vi "Update State.vi"(10 "Async Auth State":T1, 11 "Async Authorization in":refnum<class "Async Authorization.lvclass">) -> (3 "Async Authorization out":refnum<class "Async Authorization.lvclass">)   [LabVIEW 2020, in "OAuth2.lvlib" / "Async Authorization.lvclass"]
uses:
  Async Authorization.lvclass
  Async Auth State.ctl
  Async Authorization.lvclass/Async Authorization.ctl
  OAuth2.lvlib
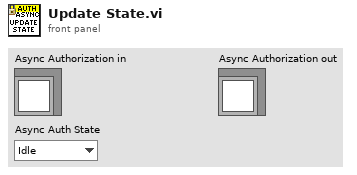
[diagram p1: front panel]
types:
  T1 = typedef "OAuth2.lvlib/Async Auth State.ctl" = enum16{"Idle", "Request", "WaitAuth", "GetToken", "RefreshToken", "Complete", "Failed"}
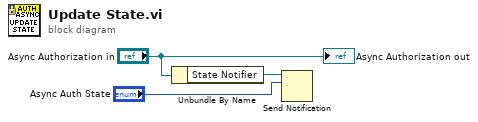
[diagram p0: block diagram]
diagram:
  n1 = Unbundle By Name("Async Authorization in") -> ("State Notifier"=w2:refnum<notifier>)
  n2 = Send Notification(notification="Async Auth State", notifier=w2) -> ()  [unwired: 1 in, 2 out]
  "Async Authorization out" <- "Async Authorization in"
